vi "ADXL345 I2C Accelerometer.vi"() -> ()   [LabVIEW 2012]
doc: "ADXL345 I2C Accelerometer\n\nThis example shows how to use the ADXL 345 Accelerometer sensor connected to I2C."
uses:
  Driver/ADXL345 I2C Range.ctl
  Driver/ADXL345 I2C Axis.ctl
  <vilib>/Rock Robotics/SystemInterfaces/Typedef/FPGA_TypedefDigitalModule.ctl
panel:
  in  "DIO Module":T1
  in  "Axis":T2 items=["X-Axis", "Y-Axis", "Z-Axis"]
  in  "Range":T3 items=["+/- 2 g", "+/- 4 g", "+/- 8 g", "+/- 16 g"]
  out "Acceleration":dbl
  out "error out":errorcluster
  in  "stop":bool
  # "Set these inputs before running."
  # "This can be set while running."
  # "Output information"
  # "Wiring Diagram for Digital Sidecar connected to an NI 9403"
  # "accelerometer"
  # "OUT"
  # "1\n2\n3\n4"
  # "5V\nSCL\nSDA\n(-)"
  # "I2C"
  # "This shows wiring for the Analog Devices ADXL345 accelerometer."
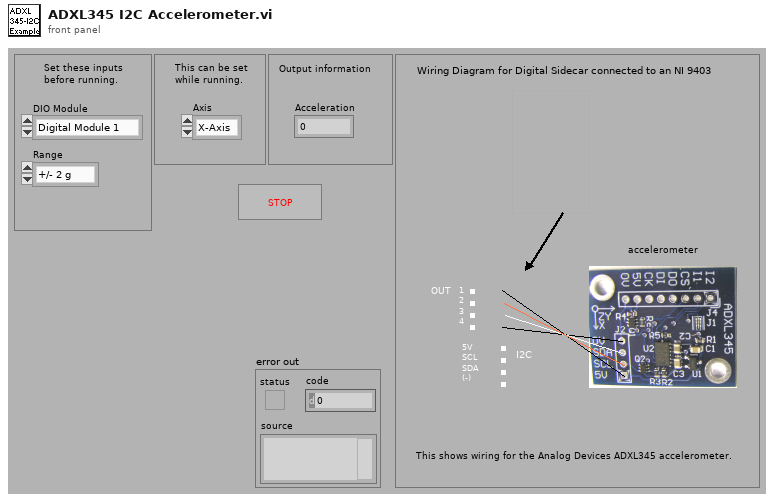
[diagram p1: front panel]
types:
  T1 = typedef "FPGA_TypedefDigitalModule.ctl" = enum16{"Digital Module 1", "Digital Module 2"}
  T2 = typedef "ADXL345 I2C Axis.ctl" = u8
  T3 = typedef "ADXL345 I2C Range.ctl" = u8
  T4 = typedef "WPI_I2CDevRef.ctl" = cluster{"DevStatus":errorcluster, "Digital Module":T1, "Device Address":u8}
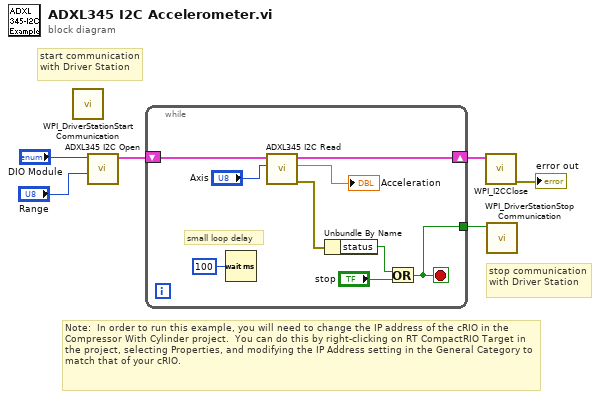
[diagram p0: block diagram]
diagram:
  # "stop communication with Driver Station"
  # "start communication with Driver Station"
  # "Note:  In order to run this example, you will need to change the IP address of the cRIO in the Compressor With Cylinder project.  You can do this by right-clicking on RT CompactRIO Target in the project, selecting Properties, and modifying the IP Address setting in the General Category to match that of your cRIO."
  n1 = call <vilib>:"WPI_DriverStationStart Communication.vi"() -> ()  [unwired: 1 in, 11 out]
  n2 = call "ADXL345 I2C Open.vi"("Range"="Range", "DIO Module (Module 1)"="DIO Module") -> ("I2CDevRef"=w6:T4)  [unwired: 2 in, 7 out]
  n3 = while {
    shift-right: [w9] -> w5
    shift-left: w6 -> [w12]
    tunnel: [w7] -> w1
    stop <- w7 stop-if-true
    # "small loop delay"
    n4 = Wait (ms)(milliseconds to wait=u32 100) -> ()  [unwired: 1 out]
    n5 = call "ADXL345 I2C Read.vi"("Axis"="Axis", "I2CDevRef"=w12) -> ("error out"=w8:errorcluster, "Acceleration"=→"Acceleration":dbl, "I2CDevRef Out"=w9:T4)  [unwired: 1 in, 6 out]
    n6 = Unbundle By Name(w8) -> ("status"=w15:bool)
    n7 = Or(x=w15, y="stop") -> (x .or. y?=w7:bool)
  }
  n8 = call <vilib>:"WPI_I2CClose.vi"("I2CDevRef"=w5) -> ("error out"=→"error out":errorcluster)  [unwired: 1 in, 9 out]
  n9 = call <vilib>:"WPI_DriverStationStop Communication.vi"("StopCommunication"=w1) -> ()  [unwired: 1 in, 10 out]
